vi "Interlock-Parameter Sweep.vi"(8 "error in (no error)":errorcluster) -> (0 "error out":errorcluster, 3 "Cancelled":bool)   [LabVIEW 2017]
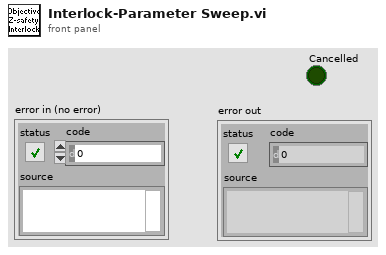
[diagram p1: front panel]
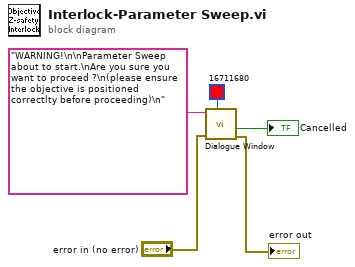
[diagram p0: block diagram]
diagram:
  n1 = call "Dialogue Window.vi"("Colour"=u32 16711680 ("Color Box"), "error in (no error)"="error in (no error)", "Message string"="WARNING!\n\nParameter Sweep about to start.\nAre you sure you want to proceed ?\n(please ensure the objective is positioned correctlty before proceeding)\n" ("message")) -> ("error out"=→"error out":errorcluster, "Cancelled (Left button pressed)"=→"Cancelled":bool)  [unwired: 6 in, 1 out]
